vi "SA Cond - Taper ALL Signals.vi"(1 "wForm IN":waveform(dbl)[](array[waveform]), 5 "error in (no error)":errorcluster, 6 "Fade Options":T1(ring), 7 "Time for Fade IN/OUT (sec)":dbl=0.25 format="%.2f", 8 "Anotate Signal Name":bool=TRUE) -> (15 "wForm OUT":waveform(dbl)[](array[waveform]), 19 "error out":errorcluster)   [LabVIEW 2020, in "GSwFormDSP.lvclass"]
uses:
  GSwFormDSP.lvclass
  Attribute List.ctl
  Attribute Options.ctl
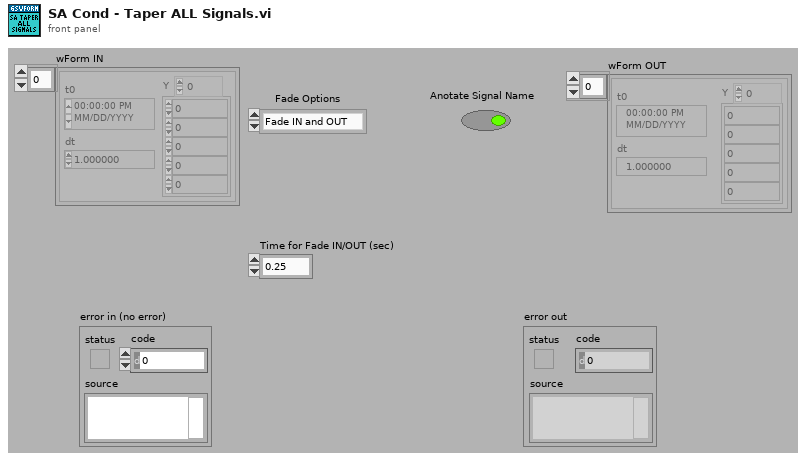
[diagram p1: front panel]
types:
  T1 = enum16{"Fade IN and OUT", "Fade IN ONLY", "Fade OUT ONLY", "None"}
  T2 = typedef "GSwFormDSP.lvclass/Attribute Options.ctl" = enum16{"Append to Attribute using \"( )\"", "Replace Attribute Value"}
  T3 = typedef "GSwFormDSP.lvclass/Attribute List.ctl" = string
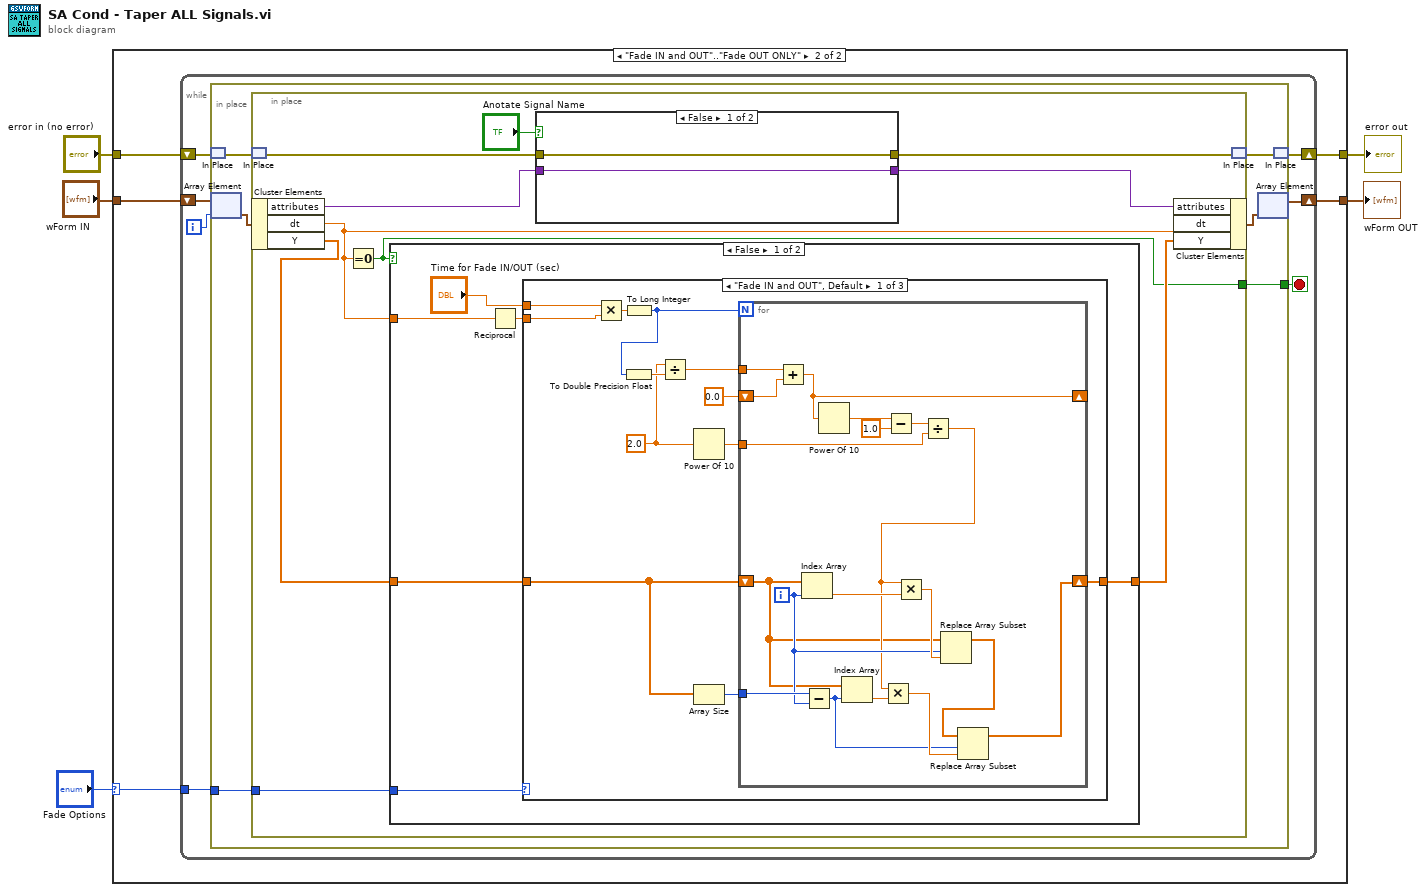
[diagram p0: block diagram]
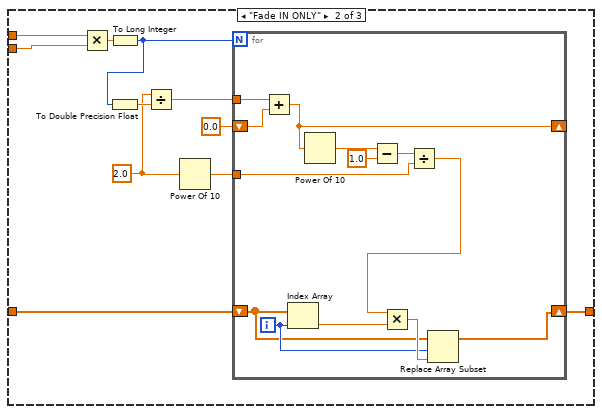
[diagram p3: hidden frame]
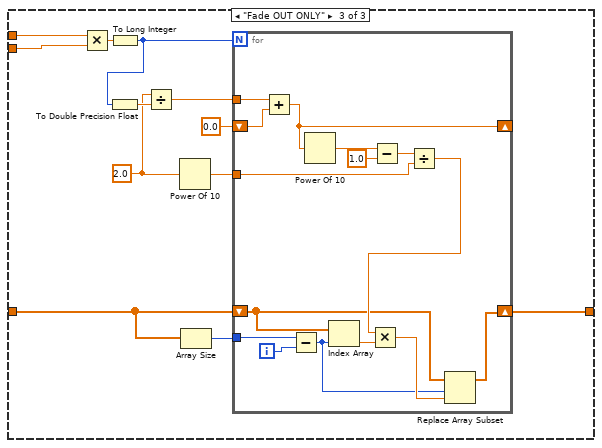
[diagram p4: hidden frame]
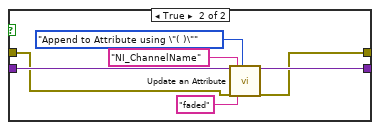
[diagram p6: hidden frame]
diagram:
  n1 = case shown="\"Fade IN and OUT\"..\"Fade OUT ONLY\"" "Fade Options" {
    selector: "Fade Options" -> [_ w12]
    tunnel: "wForm IN" -> [w7 w11]
    tunnel: [w7 w10] -> w3
    tunnel: "error in (no error)" -> [w6 w9]
    tunnel: [w6 w8] -> w1
    frame "None", Default {
    }
    frame "Fade IN and OUT".."Fade OUT ONLY" {
      n2 = while {
        shift-right: [w16] -> w10
        shift-left: w11 -> [w19]
        tunnel: w12 -> [w17]
        shift-right: [w13] -> w8
        shift-left: w9 -> [w14]
        i -> [w18]
        stop <- w15 stop-if-true
        n3 = in-place {
          in-place-border: w17 -> [w25]
          in-place-border: [w22] -> w15
          n4 = in-place-match #1(w14) -> (w21:errorcluster)
          n5 = in-place-array #2(w19, w18) -> (w24:waveform(dbl))
          n6 = in-place {
            in-place-border: w25 -> [w35]
            in-place-border: [w26] -> w22
            n7 = in-place-match #3(w21) -> (w29:errorcluster)
            n8 = in-place-cluster #4(w24) -> ("attributes"=w33:variant, "dt"=w27:dbl, "Y"=w34:dbl[])
            n9 = Equal To 0?(x=w27) -> (x = 0?=w26:bool)
            n10 = case shown="False" w26 {
              tunnel: w35 -> [w40 _]
              tunnel: w34 -> [w39 w123]
              tunnel: w27 -> [w37 _]
              tunnel: [w36 w123] -> w31
              frame False {
                n11 = Reciprocal(x=w37) -> (1/x=w38:dbl)
                n12 = case shown="\"Fade IN and OUT\", Default" w40 {
                  tunnel: w39 -> [w45 w75 w99]
                  tunnel: [w44 w74 w98] -> w36
                  tunnel: w38 -> [w43 w72 w96]
                  tunnel: "Time for Fade IN/OUT (sec)" -> [w42 w73 w97]
                  frame "Fade IN and OUT", Default {
                    w48 = 2.0
                    n13 = Multiply(x=w42, y=w43) -> (x*y=w50:dbl)
                    n14 = To Long Integer(number=w50) -> (32bit integer=w49:i32)
                    n15 = To Double Precision Float(number=w49) -> (double precision float=w53:dbl)
                    n16 = Divide(x=w48, y=w53) -> (x/y=w52:dbl)
                    n17 = Power Of 10(x=w48) -> (10^x=w47:dbl)
                    n18 = Array Size(array=w45) -> (size(s)=w46:i32)
                    n19 = for {
                      N: w49 -> [_]
                      shift-right: [w66] -> _
                      shift-left: 0.0 -> [w70]
                      tunnel: w52 -> [w71]
                      tunnel: w47 -> [w65]
                      shift-right: [w54] -> w44
                      shift-left: w45 -> [w55]
                      tunnel: w46 -> [w62]
                      i -> [w61]
                      n20 = Add(x=w71, y=w70) -> (x+y=w66:dbl)
                      n21 = Index Array(array=w55, index=w61) -> (element=w64:dbl)
                      n22 = Subtract(x=w62, y=w61) -> (x-y=w58:i32)
                      n23 = Power Of 10(x=w66) -> (10^x=w69:dbl)
                      n24 = Index Array(array=w55, index=w58) -> (element=w56:dbl)
                      n25 = Subtract(x=w69, y=1.0) -> (x-y=w68:dbl)
                      n26 = Divide(x=w68, y=w65) -> (x/y=w59:dbl)
                      n27 = Multiply(x=w59, y=w56) -> (x*y=w60:dbl)
                      n28 = Multiply(x=w59, y=w64) -> (x*y=w63:dbl)
                      n29 = Replace Array Subset(array=w55, new element=w63, index=w61) -> (w57:dbl[])
                      n30 = Replace Array Subset(array=w57, new element=w60, index=w58) -> (w54:dbl[])
                    }
                  }
                  frame "Fade IN ONLY" {
                    w77 = 2.0
                    n31 = Multiply(x=w73, y=w72) -> (x*y=w79:dbl)
                    n32 = To Long Integer(number=w79) -> (32bit integer=w78:i32)
                    n33 = To Double Precision Float(number=w78) -> (double precision float=w82:dbl)
                    n34 = Divide(x=w77, y=w82) -> (x/y=w81:dbl)
                    n35 = Power Of 10(x=w77) -> (10^x=w76:dbl)
                    n36 = for {
                      N: w78 -> [_]
                      shift-right: [w90] -> _
                      shift-left: 0.0 -> [w94]
                      tunnel: w81 -> [w95]
                      tunnel: w76 -> [w89]
                      shift-right: [w83] -> w74
                      shift-left: w75 -> [w84]
                      i -> [w86]
                      n37 = Add(x=w95, y=w94) -> (x+y=w90:dbl)
                      n38 = Index Array(array=w84, index=w86) -> (element=w88:dbl)
                      n39 = Power Of 10(x=w90) -> (10^x=w93:dbl)
                      n40 = Subtract(x=w93, y=1.0) -> (x-y=w92:dbl)
                      n41 = Divide(x=w92, y=w89) -> (x/y=w85:dbl)
                      n42 = Multiply(x=w85, y=w88) -> (x*y=w87:dbl)
                      n43 = Replace Array Subset(array=w84, new element=w87, index=w86) -> (w83:dbl[])
                    }
                  }
                  frame "Fade OUT ONLY" {
                    w102 = 2.0
                    n44 = Multiply(x=w97, y=w96) -> (x*y=w104:dbl)
                    n45 = To Long Integer(number=w104) -> (32bit integer=w103:i32)
                    n46 = To Double Precision Float(number=w103) -> (double precision float=w107:dbl)
                    n47 = Divide(x=w102, y=w107) -> (x/y=w106:dbl)
                    n48 = Power Of 10(x=w102) -> (10^x=w101:dbl)
                    n49 = Array Size(array=w99) -> (size(s)=w100:i32)
                    n50 = for {
                      N: w103 -> [_]
                      shift-right: [w117] -> _
                      shift-left: 0.0 -> [w121]
                      tunnel: w106 -> [w122]
                      tunnel: w101 -> [w116]
                      shift-right: [w109] -> w98
                      shift-left: w99 -> [w108]
                      tunnel: w100 -> [w115]
                      i -> [w114]
                      n51 = Add(x=w122, y=w121) -> (x+y=w117:dbl)
                      n52 = Subtract(x=w115, y=w114) -> (x-y=w111:i32)
                      n53 = Power Of 10(x=w117) -> (10^x=w120:dbl)
                      n54 = Index Array(array=w108, index=w111) -> (element=w110:dbl)
                      n55 = Subtract(x=w120, y=1.0) -> (x-y=w119:dbl)
                      n56 = Divide(x=w119, y=w116) -> (x/y=w112:dbl)
                      n57 = Multiply(x=w112, y=w110) -> (x*y=w113:dbl)
                      n58 = Replace Array Subset(array=w108, new element=w113, index=w111) -> (w109:dbl[])
                    }
                  }
                }
              }
              frame True {
              }
            }
            n59 = case shown="False" "Anotate Signal Name" {
              tunnel: w33 -> [w125 w132]
              tunnel: [w125 w131] -> w32
              tunnel: w29 -> [w124 w127]
              tunnel: [w124 w126] -> w28
              frame False {
              }
              frame True {
                n60 = call "Update an Attribute.vi"("attributes in"=w132, "error in (no error)"=w127, "Attribute List"=T3 "NI_ChannelName", "Attribute Value"="faded" ("string"), "Attribute Option"=Attribute_Options."Append to Attribute using \"( )\"") -> ("attributes out"=w131:variant, "error out"=w126:errorcluster)  [unwired: 13 in]
              }
            }
            n61 = in-place-cluster #4("attributes"=w32, "dt"=w27, "Y"=w31) -> (w23:waveform(dbl))
            n62 = in-place-match #3(w28) -> (w20:errorcluster)
          }
          n63 = in-place-array #2(w23) -> (w16:waveform(dbl)[])  [unwired: 1 out]
          n64 = in-place-match #1(w20) -> (w13:errorcluster)
        }
      }
    }
  }
  "wForm OUT" <- w3
  "error out" <- w1
